vi "Load LVS.vi"(8 "error in (no error)":errorcluster, 10 "LVS Data (in)":T1={"Impulse Positions"=[], "No. Imp"=0, "Parameter Time Series"=[], "Parameter Impuls Series"=[], "Experiment Parameters"={"Freq"=0.0, "Vel"=0, "Acc"=0, "Stimulus"=""}, "Autosort File"=refnum, "Data File"={"Data Channels"=[], "Sample Rate"=0, "Channel List"=[]}, "Experiment data path"=path "/Macintosh HD/Users/patrick/Studium/Diploma Thesis/Data Analysis", "Image data path"=path "/Macintosh HD/Users/patrick/Studium/Diploma Thesis/Data Analysis", "LVS data path"=path "/Macintosh HD/Users/patrick/Studium/Diploma Thesis/Data Analysis", "Raw copy path"=path "/Macintosh HD/Users/patrick/Studium/Diploma Thesis/Data Analysis", "filename"="No file selected", "desaccading parameters"={"Tolerance"=0, "Acc Range"=0.0, "Sample Rate"=0, "Impulse Plane 2"=enum."Other", "Impulse dir"=FALSE}, "Experiment Parameters 2"={"Subject"="", "Strain"="", "Rotation plane"="", "Experimenter"="", "Trial"=0.0, "Time"=0.0}, "Excel"={"Excel._Application"=refnum, "Use Excel"=FALSE, "Worksheet SINE"=refnum, "Row SINE"=0, "Worksheet TRANS"=refnum, "Row TRANS"=0}, "Session Config File"=refnum, "Autosort Parameter Set"=1, "EMA Version"="", "desacc "={"Threshold 1 [Acc]"=7000.0, "Threshold 2 [% of TH1]"=60, "tolerance"=3, "Search WD "=0.1, " always use TH2"=FALSE, "Range"=2.0, "Max time"=120.0, "Min time"=20.0, "Velocity Threshold"=150}, "Cycle Nr for Saccades"={"POS"=0, "NEG"=0}, "calibration name"="No file selected"} {"Parameter Time Series"."time offset" format="%.3f"; "Parameter Time Series"."Gain" format="%.1f"; "Parameter Time Series"."Offset" format="%.1f"; "Parameter Time Series"."List 1" items=["Motor-Pos", "Motor-Vel", "Lx Position-in-Head", "Ly Position-in-Head", "Lz Position-in-Head", "Lx Velocity-in-Head", "Ly Velocity-in-Head", "Lz Velocity-in-Head", "Ll Velocity-in-Head", "Lr Velocity-in-Head", "Lx Accel-in-Head", "Ly Accel-in-Head", "Lz Accel-in-Head", "Rx Position-in-Head", "Ry Position-in-Head", "Rz Position-in-Head", "Rx Velocity-in-Head", "Ry Velocity-in-Head", "Rz Velocity-in-Head", "Rl Velocity-in-Head", "Rr Velocity-in-Head", "Rx Accel-in-Head", "Ry Accel-in-Head", "Rz Accel-in-Head", "Global Trigger", "", "", ""]; "Parameter Impuls Series"."Gain" format="%.1f"; "Parameter Impuls Series"."Offset" format="%.1f"}, 11 "Path (in)":path) -> (0 "error out":errorcluster, 2 "LVS Data (out)":T1={"Impulse Positions"=[], "No. Imp"=0, "Parameter Time Series"=[], "Parameter Impuls Series"=[], "Experiment Parameters"={"Freq"=0.0, "Vel"=0, "Acc"=0, "Stimulus"=""}, "Autosort File"=refnum, "Data File"={"Data Channels"=[], "Sample Rate"=0, "Channel List"=[]}, "Experiment data path"=path "/Macintosh HD/Users/patrick/Studium/Diploma Thesis/Data Analysis", "Image data path"=path "/Macintosh HD/Users/patrick/Studium/Diploma Thesis/Data Analysis", "LVS data path"=path "/Macintosh HD/Users/patrick/Studium/Diploma Thesis/Data Analysis", "Raw copy path"=path "/Macintosh HD/Users/patrick/Studium/Diploma Thesis/Data Analysis", "filename"="No file selected", "desaccading parameters"={"Tolerance"=0, "Acc Range"=0.0, "Sample Rate"=0, "Impulse Plane 2"=enum."Other", "Impulse dir"=FALSE}, "Experiment Parameters 2"={"Subject"="", "Strain"="", "Rotation plane"="", "Experimenter"="", "Trial"=0.0, "Time"=0.0}, "Excel"={"Excel._Application"=refnum, "Use Excel"=FALSE, "Worksheet SINE"=refnum, "Row SINE"=0, "Worksheet TRANS"=refnum, "Row TRANS"=0}, "Session Config File"=refnum, "Autosort Parameter Set"=1, "EMA Version"="", "desacc "={"Threshold 1 [Acc]"=7000.0, "Threshold 2 [% of TH1]"=60, "tolerance"=3, "Search WD "=0.1, " always use TH2"=FALSE, "Range"=2.0, "Max time"=120.0, "Min time"=20.0, "Velocity Threshold"=150}, "Cycle Nr for Saccades"={"POS"=0, "NEG"=0}, "calibration name"="No file selected"} {"Parameter Time Series"."time offset" format="%.3f"; "Parameter Time Series"."Gain" format="%.1f"; "Parameter Time Series"."Offset" format="%.1f"; "Parameter Time Series"."List 1" items=["Motor-Pos", "Motor-Vel", "Lx Position-in-Head", "Ly Position-in-Head", "Lz Position-in-Head", "Lx Velocity-in-Head", "Ly Velocity-in-Head", "Lz Velocity-in-Head", "Ll Velocity-in-Head", "Lr Velocity-in-Head", "Lx Accel-in-Head", "Ly Accel-in-Head", "Lz Accel-in-Head", "Rx Position-in-Head", "Ry Position-in-Head", "Rz Position-in-Head", "Rx Velocity-in-Head", "Ry Velocity-in-Head", "Rz Velocity-in-Head", "Rl Velocity-in-Head", "Rr Velocity-in-Head", "Rx Accel-in-Head", "Ry Accel-in-Head", "Rz Accel-in-Head", "Global Trigger", "", "", ""]; "Parameter Impuls Series"."Gain" format="%.1f"; "Parameter Impuls Series"."Offset" format="%.1f"}, 3 "Path (out)":path)   [LabVIEW 2016]
uses:
  type-defs/TD_Statemachine-Data.ctl
  type-defs/TD_Time Series.ctl
  type-defs/TD_Impulse Parameter.ctl
  core.lvlib
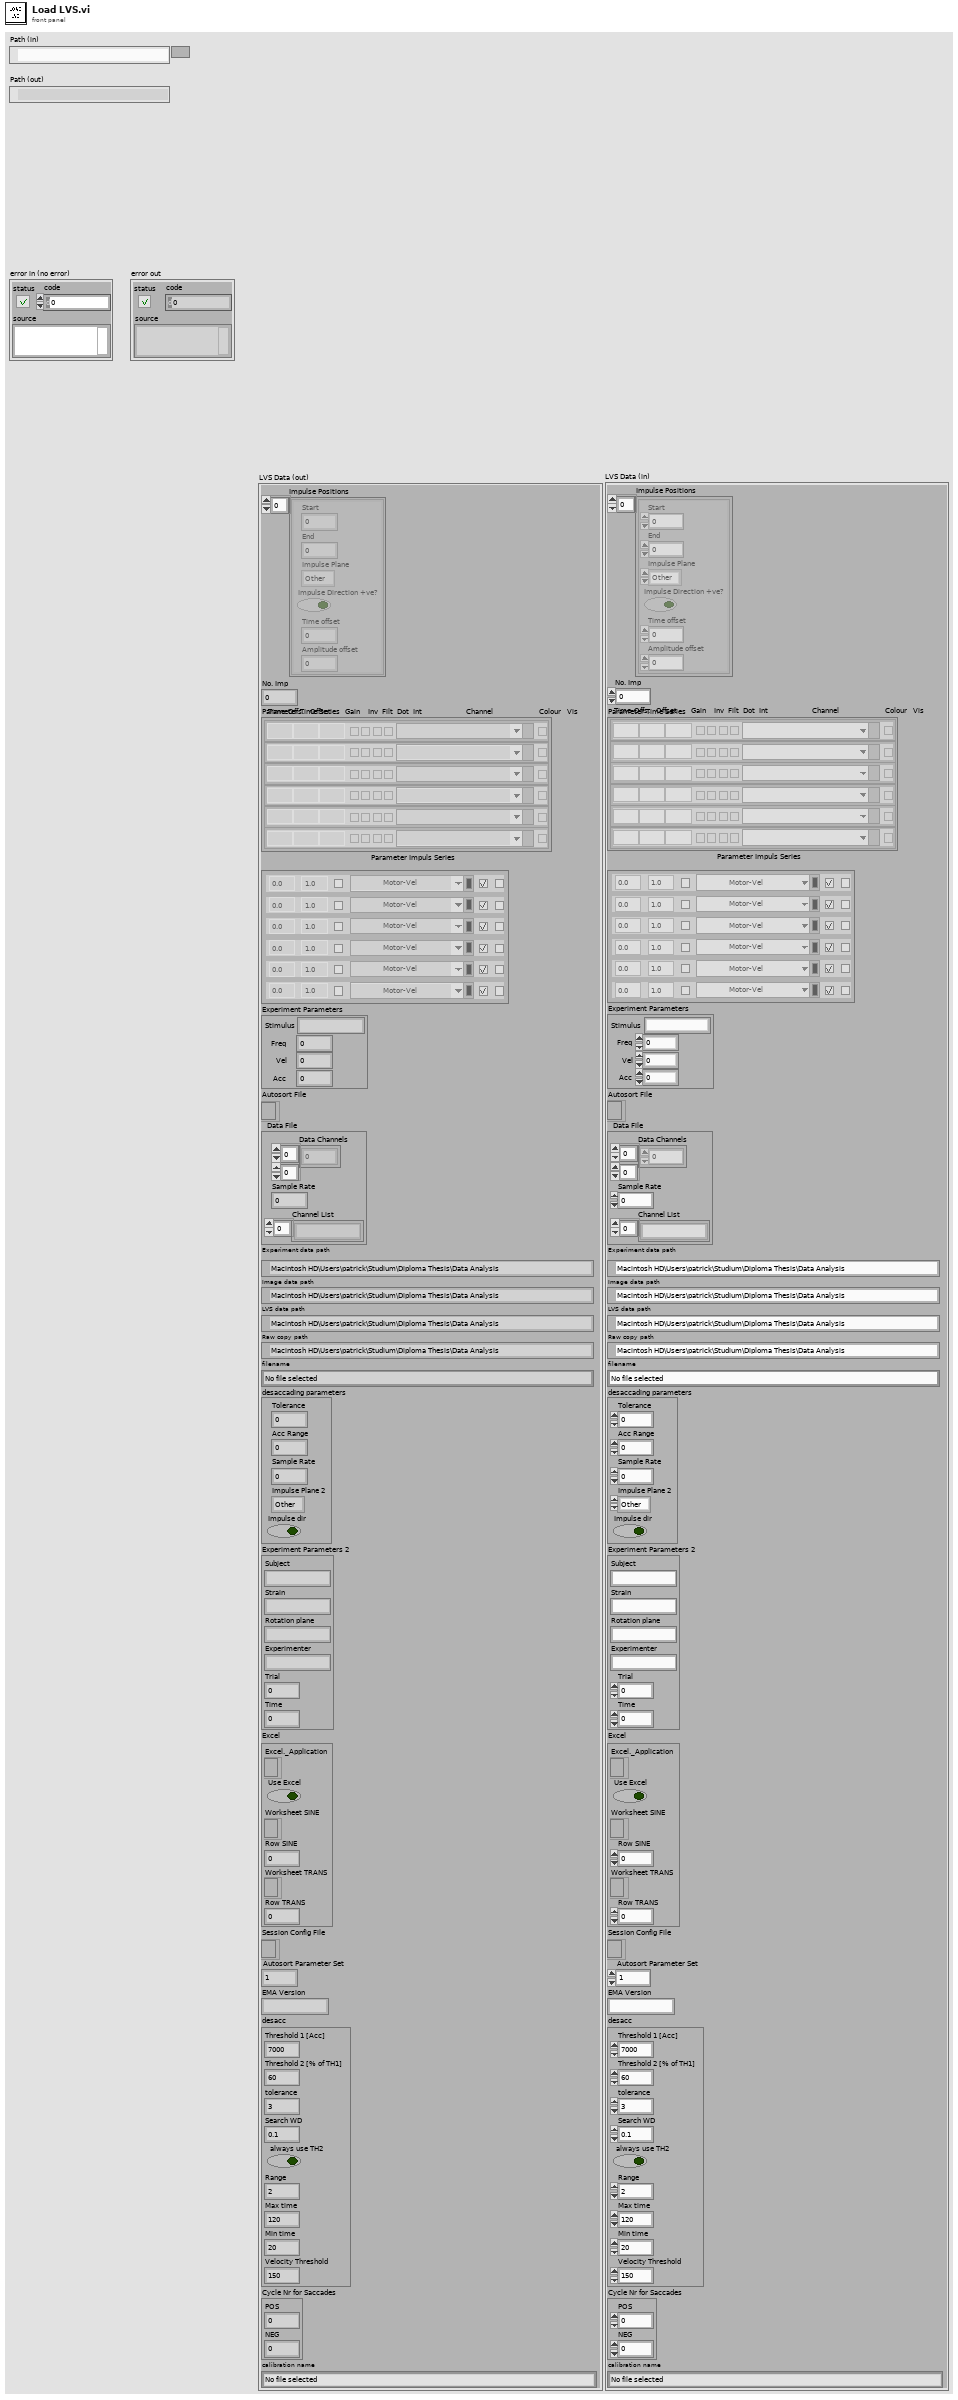
[diagram p1: front panel]
types:
  T1 = typedef "core.lvlib/TD_Statemachine-Data.ctl" = cluster{"Impulse Positions":cluster{"Start":i32, "End":i32, "Impulse Plane":enum16{"Other", "Yaw", "Pitch", "Roll", "LARP", "RALP"}, "Impulse Direction +ve?":bool, "Time offset":i32, "Amplitude offset":dbl}[], "No. Imp":i32, "Parameter Time Series":T2, "Parameter Impuls Series":T3, "Experiment Parameters":cluster{"Freq":dbl, "Vel":i32, "Acc":i32, "Stimulus":string}, "Autosort File":refnum<file>, "Data File":cluster{"Data Channels":dbl[][], "Sample Rate":i32, "Channel List":string[]}, "Experiment data path":path, "Image data path":path, "LVS data path":path, "Raw copy path":path, "filename":string, "desaccading parameters":cluster{"Tolerance":i32, "Acc Range":dbl, "Sample Rate":i32, "Impulse Plane 2":enum16{"Other", "Yaw", "Pitch", "Roll", "LARP", "RALP"}, "Impulse dir":bool}, "Experiment Parameters 2":cluster{"Subject":string, "Strain":string, "Rotation plane":string, "Experimenter":string, "Trial":dbl, "Time":dbl}, "Excel":cluster{"Excel._Application":refnum<k7>, "Use Excel":bool, "Worksheet SINE":refnum<k7>, "Row SINE":i32, "Worksheet TRANS":refnum<k7>, "Row TRANS":i32}, "Session Config File":refnum<file>, "Autosort Parameter Set":i32, "EMA Version":string, "desacc ":cluster{"Threshold 1 [Acc]":dbl, "Threshold 2 [% of TH1]":i32, "tolerance":i32, "Search WD ":dbl, " always use TH2":bool, "Range":dbl, "Max time":dbl, "Min time":dbl, "Velocity Threshold":i32}, "Cycle Nr for Saccades":cluster{"POS":i32, "NEG":i32}, "calibration name":string}
  T2 = typedef "core.lvlib/TD_Time Series.ctl" = cluster{"time offset":dbl, "Offset":dbl, "Gain":dbl, "inverse":bool, "filter data":bool, "dots":bool, "interpolate":bool, "List 1":u16, "Color Box":u32, "Boolean":bool}[]
  T3 = typedef "core.lvlib/TD_Impulse Parameter.ctl" = cluster{"Color":u32, "Visible":bool, "Channel":u16, "Invert":bool, "Desaccade":bool, "Offset":dbl, "Gain":dbl}[]
  T4 = cluster{"Data Channels":dbl[][], "Sample Rate":i32, "Channel List":string[]}
  T5 = cluster{"Freq":dbl, "Vel":i32, "Acc":i32, "Stimulus":string}
  T6 = cluster{"Subject":string, "Strain":string, "Rotation plane":string, "Experimenter":string, "Trial":dbl, "Time":dbl}
  T7 = cluster{"Impulse Positions":cluster{"Start":i32, "End":i32, "Impulse Plane":enum16{"Other", "Yaw", "Pitch", "Roll", "LARP", "RALP"}, "Impulse Direction +ve?":bool, "Time offset":i32, "Amplitude offset":dbl}[], "Old Impulse positions for Undo":cluster{"Start":i32, "End":i32, "Impulse Plane":enum16{"Other", "Yaw", "Pitch", "Roll", "LARP", "RALP"}, "Impulse Direction +ve?":bool, "Time offset":i32, "Amplitude offset":dbl}[], "No. Imp":i32}
  T8 = cluster{"\"Data File\" Cluster":cluster{"Data Channels":dbl[][], "Sample Rate":i32, "Channel List":string[]}, "OLD LVS Data Cluster":cluster{"Impulse Positions":cluster{"Start":i32, "End":i32, "Impulse Plane":enum16{"Other", "Yaw", "Pitch", "Roll", "LARP", "RALP"}, "Impulse Direction +ve?":bool, "Time offset":i32, "Amplitude offset":dbl}[], "Old Impulse positions for Undo":cluster{"Start":i32, "End":i32, "Impulse Plane":enum16{"Other", "Yaw", "Pitch", "Roll", "LARP", "RALP"}, "Impulse Direction +ve?":bool, "Time offset":i32, "Amplitude offset":dbl}[], "No. Imp":i32}}
  T9 = cluster{"Start":i32, "End":i32, "Impulse Plane":enum16{"Other", "Yaw", "Pitch", "Roll", "LARP", "RALP"}, "Impulse Direction +ve?":bool, "Time offset":i32, "Amplitude offset":dbl}[]
  T10 = cluster{"Impulse Positions":cluster{"Start":i32, "End":i32, "Impulse Plane":enum16{"Other", "Yaw", "Pitch", "Roll", "LARP", "RALP"}, "Impulse Direction +ve?":bool, "Time offset":i32, "Amplitude offset":dbl}[], "Old Impulse positions for Undo":cluster{"Start":i32, "End":i32, "Impulse Plane":enum16{"Other", "Yaw", "Pitch", "Roll", "LARP", "RALP"}, "Impulse Direction +ve?":bool, "Time offset":i32, "Amplitude offset":dbl}[], "No. Imp":i32, "Parameter Time Series":T2, "Parameter Impuls Series":T3, "Experiment Parameters":cluster{"Freq":dbl, "Vel":i32, "Acc":i32, "Stimulus":string}, "Autosort File":refnum<file>, "Data File":cluster{"Data Channels":dbl[][], "Sample Rate":i32, "Channel List":string[]}, "Experiment data path":path, "Image data path":path, "LVS data path":path, "Raw copy path":path, "filename":string, "desaccading parameters":cluster{"Tolerance":i32, "Acc Range":dbl, "Sample Rate":i32, "Impulse Plane 2":enum16{"Other", "Yaw", "Pitch", "Roll", "LARP", "RALP"}, "Impulse dir":bool}, "Experiment Parameters 2":cluster{"Subject":string, "Strain":string, "Rotation plane":string, "Experimenter":string, "Trial":dbl, "Time":dbl}, "Excel":cluster{"Excel._Application":refnum<k7>, "Use Excel":bool, "Worksheet SINE":refnum<k7>, "Row SINE":i32, "Worksheet TRANS":refnum<k7>, "Row TRANS":i32}, "Session Config File":refnum<file>, "Autosort Parameter Set":i32, "EMA Version":string, "desacc ":cluster{"Threshold 1 [Acc]":dbl, "Threshold 2 [% of TH1]":i32, "tolerance":i32, "Search WD ":dbl, " always use TH2":bool, "Range":dbl, "Max time":dbl, "Min time":dbl}}
  T11 = cluster{"\"Data File\" Cluster":cluster{"Data Channels":dbl[][], "Sample Rate":i32, "Channel List":string[]}, "EMA 2011a Data Cluster":cluster{"Impulse Positions":cluster{"Start":i32, "End":i32, "Impulse Plane":enum16{"Other", "Yaw", "Pitch", "Roll", "LARP", "RALP"}, "Impulse Direction +ve?":bool, "Time offset":i32, "Amplitude offset":dbl}[], "Old Impulse positions for Undo":cluster{"Start":i32, "End":i32, "Impulse Plane":enum16{"Other", "Yaw", "Pitch", "Roll", "LARP", "RALP"}, "Impulse Direction +ve?":bool, "Time offset":i32, "Amplitude offset":dbl}[], "No. Imp":i32, "Parameter Time Series":T2, "Parameter Impuls Series":T3, "Experiment Parameters":cluster{"Freq":dbl, "Vel":i32, "Acc":i32, "Stimulus":string}, "Autosort File":refnum<file>, "Data File":cluster{"Data Channels":dbl[][], "Sample Rate":i32, "Channel List":string[]}, "Experiment data path":path, "Image data path":path, "LVS data path":path, "Raw copy path":path, "filename":string, "desaccading parameters":cluster{"Tolerance":i32, "Acc Range":dbl, "Sample Rate":i32, "Impulse Plane 2":enum16{"Other", "Yaw", "Pitch", "Roll", "LARP", "RALP"}, "Impulse dir":bool}, "Experiment Parameters 2":cluster{"Subject":string, "Strain":string, "Rotation plane":string, "Experimenter":string, "Trial":dbl, "Time":dbl}, "Excel":cluster{"Excel._Application":refnum<k7>, "Use Excel":bool, "Worksheet SINE":refnum<k7>, "Row SINE":i32, "Worksheet TRANS":refnum<k7>, "Row TRANS":i32}, "Session Config File":refnum<file>, "Autosort Parameter Set":i32, "EMA Version":string, "desacc ":cluster{"Threshold 1 [Acc]":dbl, "Threshold 2 [% of TH1]":i32, "tolerance":i32, "Search WD ":dbl, " always use TH2":bool, "Range":dbl, "Max time":dbl, "Min time":dbl}}}
  T12 = cluster{"Tolerance":i32, "Acc Range":dbl, "Sample Rate":i32, "Impulse Plane 2":enum16{"Other", "Yaw", "Pitch", "Roll", "LARP", "RALP"}, "Impulse dir":bool}
  T13 = cluster{"Impulse Positions":cluster{"Start":i32, "End":i32, "Impulse Plane":enum16{"Other", "Yaw", "Pitch", "Roll", "LARP", "RALP"}, "Impulse Direction +ve?":bool, "Time offset":i32, "Amplitude offset":dbl}[], "Old Impulse positions for Undo":cluster{"Start":i32, "End":i32, "Impulse Plane":enum16{"Other", "Yaw", "Pitch", "Roll", "LARP", "RALP"}, "Impulse Direction +ve?":bool, "Time offset":i32, "Amplitude offset":dbl}[][], "No. Imp":i32, "Parameter Time Series":T2, "Parameter Impuls Series":T3, "Experiment Parameters":cluster{"Freq":dbl, "Vel":i32, "Acc":i32, "Stimulus":string}, "Autosort File":refnum<file>, "Data File":cluster{"Data Channels":dbl[][], "Sample Rate":i32, "Channel List":string[]}, "Experiment data path":path, "Image data path":path, "LVS data path":path, "Raw copy path":path, "filename":string, "desaccading parameters":cluster{"Tolerance":i32, "Acc Range":dbl, "Sample Rate":i32, "Impulse Plane 2":enum16{"Other", "Yaw", "Pitch", "Roll", "LARP", "RALP"}, "Impulse dir":bool}, "Experiment Parameters 2":cluster{"Subject":string, "Strain":string, "Rotation plane":string, "Experimenter":string, "Trial":dbl, "Time":dbl}, "Excel":cluster{"Excel._Application":refnum<k7>, "Use Excel":bool, "Worksheet SINE":refnum<k7>, "Row SINE":i32, "Worksheet TRANS":refnum<k7>, "Row TRANS":i32}, "Session Config File":refnum<file>, "Autosort Parameter Set":i32, "EMA Version":string, "desacc ":cluster{"Threshold 1 [Acc]":dbl, "Threshold 2 [% of TH1]":i32, "tolerance":i32, "Search WD ":dbl, " always use TH2":bool, "Range":dbl, "Max time":dbl, "Min time":dbl, "Velocity Threshold":i32}, "Cycle Nr for Saccades":cluster{"POS":i32, "NEG":i32}, "Undo Counter":i32, "History Length":i32, "Redo Counter":i32, "Histpry Position":i32, "Raw Data File":cluster{"Data Channels":dbl[][], "Sample Rate":i32, "Channel List":string[]}}
  T14 = cluster{"\"Data File\" Cluster":cluster{"Data Channels":dbl[][], "Sample Rate":i32, "Channel List":string[]}, "EMA 2011b Data Cluster":cluster{"Impulse Positions":cluster{"Start":i32, "End":i32, "Impulse Plane":enum16{"Other", "Yaw", "Pitch", "Roll", "LARP", "RALP"}, "Impulse Direction +ve?":bool, "Time offset":i32, "Amplitude offset":dbl}[], "Old Impulse positions for Undo":cluster{"Start":i32, "End":i32, "Impulse Plane":enum16{"Other", "Yaw", "Pitch", "Roll", "LARP", "RALP"}, "Impulse Direction +ve?":bool, "Time offset":i32, "Amplitude offset":dbl}[][], "No. Imp":i32, "Parameter Time Series":T2, "Parameter Impuls Series":T3, "Experiment Parameters":cluster{"Freq":dbl, "Vel":i32, "Acc":i32, "Stimulus":string}, "Autosort File":refnum<file>, "Data File":cluster{"Data Channels":dbl[][], "Sample Rate":i32, "Channel List":string[]}, "Experiment data path":path, "Image data path":path, "LVS data path":path, "Raw copy path":path, "filename":string, "desaccading parameters":cluster{"Tolerance":i32, "Acc Range":dbl, "Sample Rate":i32, "Impulse Plane 2":enum16{"Other", "Yaw", "Pitch", "Roll", "LARP", "RALP"}, "Impulse dir":bool}, "Experiment Parameters 2":cluster{"Subject":string, "Strain":string, "Rotation plane":string, "Experimenter":string, "Trial":dbl, "Time":dbl}, "Excel":cluster{"Excel._Application":refnum<k7>, "Use Excel":bool, "Worksheet SINE":refnum<k7>, "Row SINE":i32, "Worksheet TRANS":refnum<k7>, "Row TRANS":i32}, "Session Config File":refnum<file>, "Autosort Parameter Set":i32, "EMA Version":string, "desacc ":cluster{"Threshold 1 [Acc]":dbl, "Threshold 2 [% of TH1]":i32, "tolerance":i32, "Search WD ":dbl, " always use TH2":bool, "Range":dbl, "Max time":dbl, "Min time":dbl, "Velocity Threshold":i32}, "Cycle Nr for Saccades":cluster{"POS":i32, "NEG":i32}, "Undo Counter":i32, "History Length":i32, "Redo Counter":i32, "Histpry Position":i32, "Raw Data File":cluster{"Data Channels":dbl[][], "Sample Rate":i32, "Channel List":string[]}}}
  T15 = cluster{"Threshold 1 [Acc]":dbl, "Threshold 2 [% of TH1]":i32, "tolerance":i32, "Search WD ":dbl, " always use TH2":bool, "Range":dbl, "Max time":dbl, "Min time":dbl, "Velocity Threshold":i32}
  T16 = cluster{"Impulse Positions":cluster{"Start":i32, "End":i32, "Impulse Plane":enum16{"Other", "Yaw", "Pitch", "Roll", "LARP", "RALP"}, "Impulse Direction +ve?":bool, "Time offset":i32, "Amplitude offset":dbl}[], "Old Impulse positions for Undo":cluster{"Start":i32, "End":i32, "Impulse Plane":enum16{"Other", "Yaw", "Pitch", "Roll", "LARP", "RALP"}, "Impulse Direction +ve?":bool, "Time offset":i32, "Amplitude offset":dbl}[][], "No. Imp":i32, "Parameter Time Series":T2, "Parameter Impuls Series":T3, "Experiment Parameters":cluster{"Freq":dbl, "Vel":i32, "Acc":i32, "Stimulus":string}, "Autosort File":refnum<file>, "Data File":cluster{"Data Channels":dbl[][], "Sample Rate":i32, "Channel List":string[]}, "Experiment data path":path, "Image data path":path, "LVS data path":path, "Raw copy path":path, "filename":string, "desaccading parameters":cluster{"Tolerance":i32, "Acc Range":dbl, "Sample Rate":i32, "Impulse Plane 2":enum16{"Other", "Yaw", "Pitch", "Roll", "LARP", "RALP"}, "Impulse dir":bool}, "Experiment Parameters 2":cluster{"Subject":string, "Strain":string, "Rotation plane":string, "Experimenter":string, "Trial":dbl, "Time":dbl}, "Excel":cluster{"Excel._Application":refnum<k7>, "Use Excel":bool, "Worksheet SINE":refnum<k7>, "Row SINE":i32, "Worksheet TRANS":refnum<k7>, "Row TRANS":i32}, "Session Config File":refnum<file>, "Autosort Parameter Set":i32, "EMA Version":string, "desacc ":cluster{"Threshold 1 [Acc]":dbl, "Threshold 2 [% of TH1]":i32, "tolerance":i32, "Search WD ":dbl, " always use TH2":bool, "Range":dbl, "Max time":dbl, "Min time":dbl, "Velocity Threshold":i32}, "Cycle Nr for Saccades":cluster{"POS":i32, "NEG":i32}, "Undo Counter":i32, "History Length":i32, "Redo Counter":i32, "Histpry Position":i32, "Raw Data File":cluster{"Data Channels":dbl[][], "Sample Rate":i32, "Channel List":string[]}, "calibration name":string}
  T17 = cluster{"\"Data File\" Cluster":cluster{"Data Channels":dbl[][], "Sample Rate":i32, "Channel List":string[]}, "EMA 2016a Data Cluster":cluster{"Impulse Positions":cluster{"Start":i32, "End":i32, "Impulse Plane":enum16{"Other", "Yaw", "Pitch", "Roll", "LARP", "RALP"}, "Impulse Direction +ve?":bool, "Time offset":i32, "Amplitude offset":dbl}[], "Old Impulse positions for Undo":cluster{"Start":i32, "End":i32, "Impulse Plane":enum16{"Other", "Yaw", "Pitch", "Roll", "LARP", "RALP"}, "Impulse Direction +ve?":bool, "Time offset":i32, "Amplitude offset":dbl}[][], "No. Imp":i32, "Parameter Time Series":T2, "Parameter Impuls Series":T3, "Experiment Parameters":cluster{"Freq":dbl, "Vel":i32, "Acc":i32, "Stimulus":string}, "Autosort File":refnum<file>, "Data File":cluster{"Data Channels":dbl[][], "Sample Rate":i32, "Channel List":string[]}, "Experiment data path":path, "Image data path":path, "LVS data path":path, "Raw copy path":path, "filename":string, "desaccading parameters":cluster{"Tolerance":i32, "Acc Range":dbl, "Sample Rate":i32, "Impulse Plane 2":enum16{"Other", "Yaw", "Pitch", "Roll", "LARP", "RALP"}, "Impulse dir":bool}, "Experiment Parameters 2":cluster{"Subject":string, "Strain":string, "Rotation plane":string, "Experimenter":string, "Trial":dbl, "Time":dbl}, "Excel":cluster{"Excel._Application":refnum<k7>, "Use Excel":bool, "Worksheet SINE":refnum<k7>, "Row SINE":i32, "Worksheet TRANS":refnum<k7>, "Row TRANS":i32}, "Session Config File":refnum<file>, "Autosort Parameter Set":i32, "EMA Version":string, "desacc ":cluster{"Threshold 1 [Acc]":dbl, "Threshold 2 [% of TH1]":i32, "tolerance":i32, "Search WD ":dbl, " always use TH2":bool, "Range":dbl, "Max time":dbl, "Min time":dbl, "Velocity Threshold":i32}, "Cycle Nr for Saccades":cluster{"POS":i32, "NEG":i32}, "Undo Counter":i32, "History Length":i32, "Redo Counter":i32, "Histpry Position":i32, "Raw Data File":cluster{"Data Channels":dbl[][], "Sample Rate":i32, "Channel List":string[]}, "calibration name":string}}
  T18 = cluster{"Impulse Positions":cluster{"Start":i32, "End":i32, "Impulse Plane":enum16{"Other", "Yaw", "Pitch", "Roll", "LARP", "RALP"}, "Impulse Direction +ve?":bool, "Time offset":i32, "Amplitude offset":dbl}[], "No. Imp":i32, "Parameter Time Series":T2, "Parameter Impuls Series":T3, "Experiment Parameters":cluster{"Freq":dbl, "Vel":i32, "Acc":i32, "Stimulus":string}, "Autosort File":refnum<file>, "Data File":cluster{"Data Channels":dbl[][], "Sample Rate":i32, "Channel List":string[]}, "Experiment data path":path, "Image data path":path, "LVS data path":path, "Raw copy path":path, "filename":string, "desaccading parameters":cluster{"Tolerance":i32, "Acc Range":dbl, "Sample Rate":i32, "Impulse Plane 2":enum16{"Other", "Yaw", "Pitch", "Roll", "LARP", "RALP"}, "Impulse dir":bool}, "Experiment Parameters 2":cluster{"Subject":string, "Strain":string, "Rotation plane":string, "Experimenter":string, "Trial":dbl, "Time":dbl}, "Excel":cluster{"Excel._Application":refnum<k7>, "Use Excel":bool, "Worksheet SINE":refnum<k7>, "Row SINE":i32, "Worksheet TRANS":refnum<k7>, "Row TRANS":i32}, "Session Config File":refnum<file>, "Autosort Parameter Set":i32, "EMA Version":string, "desacc ":cluster{"Threshold 1 [Acc]":dbl, "Threshold 2 [% of TH1]":i32, "tolerance":i32, "Search WD ":dbl, " always use TH2":bool, "Range":dbl, "Max time":dbl, "Min time":dbl, "Velocity Threshold":i32}, "Cycle Nr for Saccades":cluster{"POS":i32, "NEG":i32}, "calibration name":string}
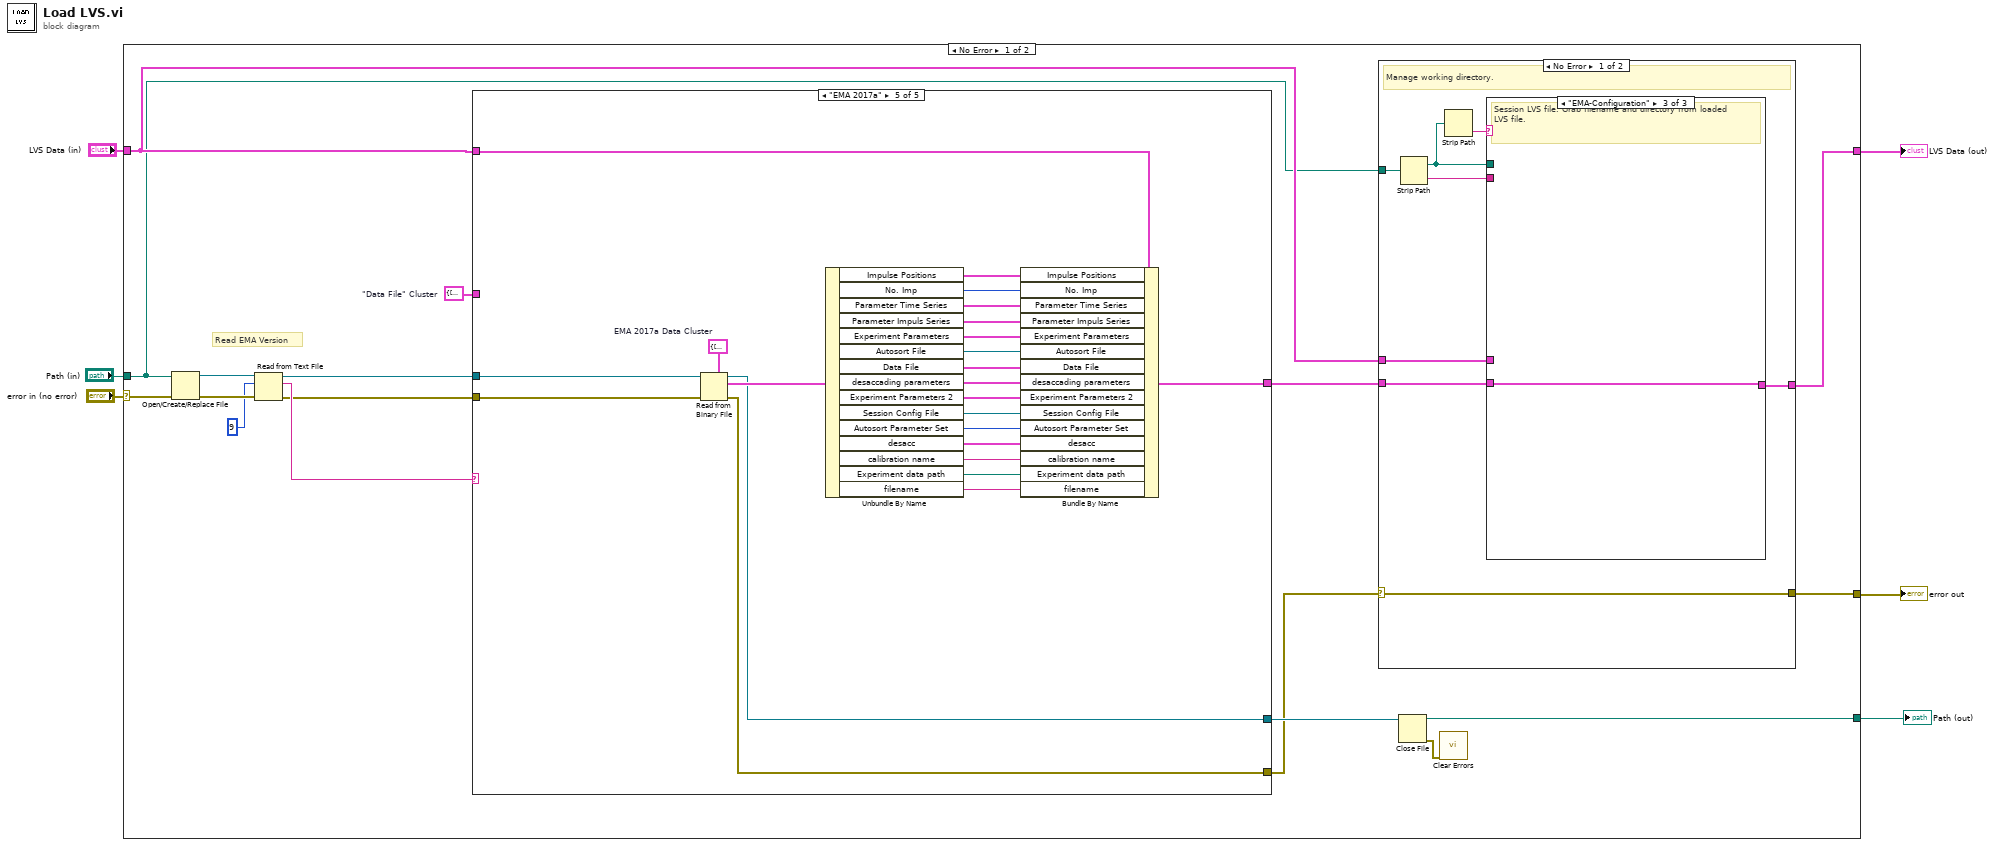
[diagram p0: block diagram]
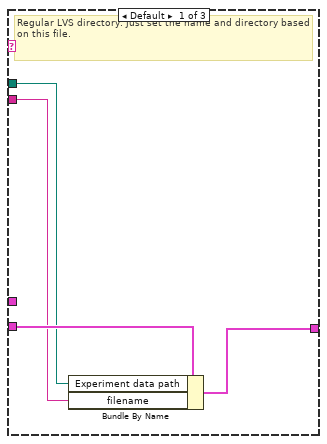
[diagram p2: hidden frame]
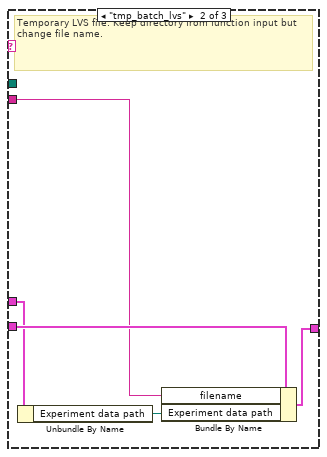
[diagram p3: hidden frame]
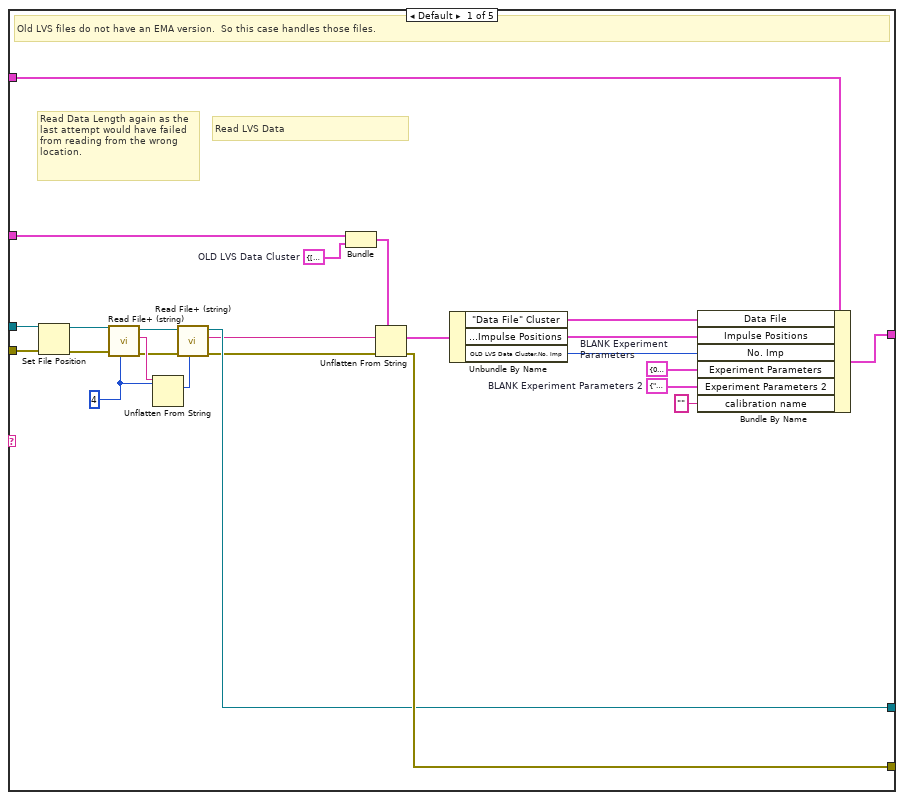
[diagram p5: hidden frame]
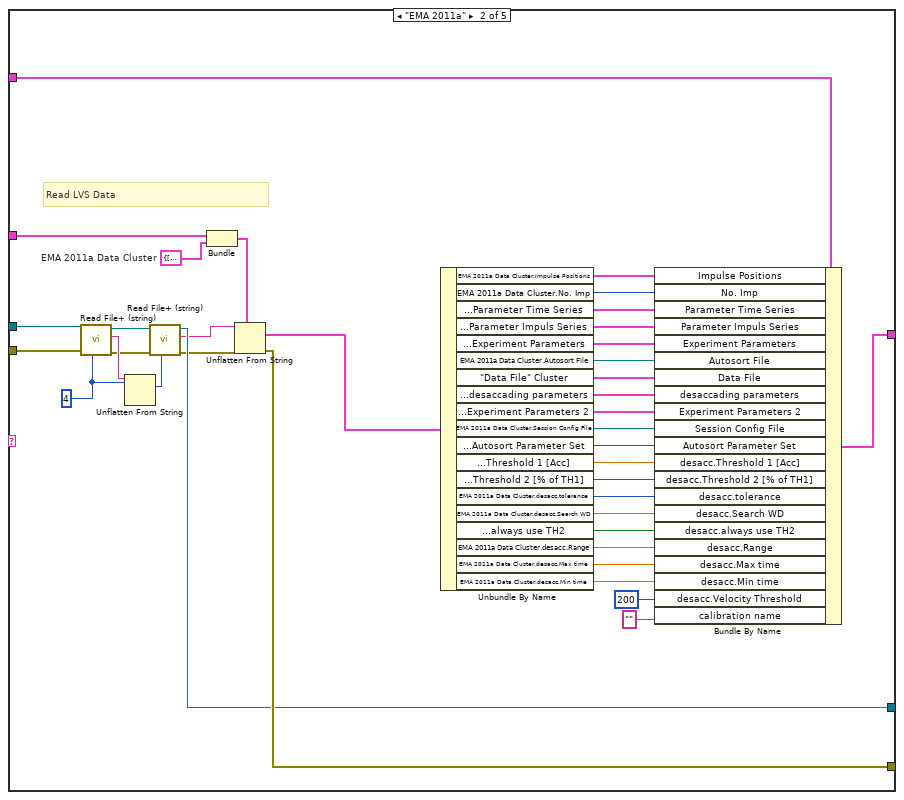
[diagram p6: hidden frame]
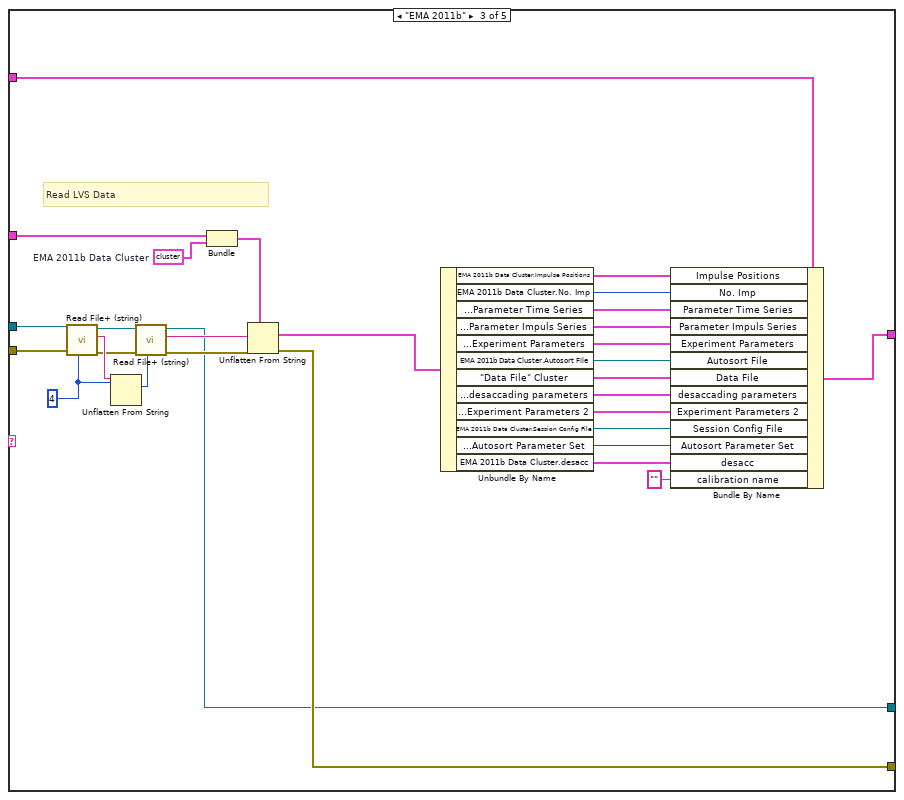
[diagram p7: hidden frame]
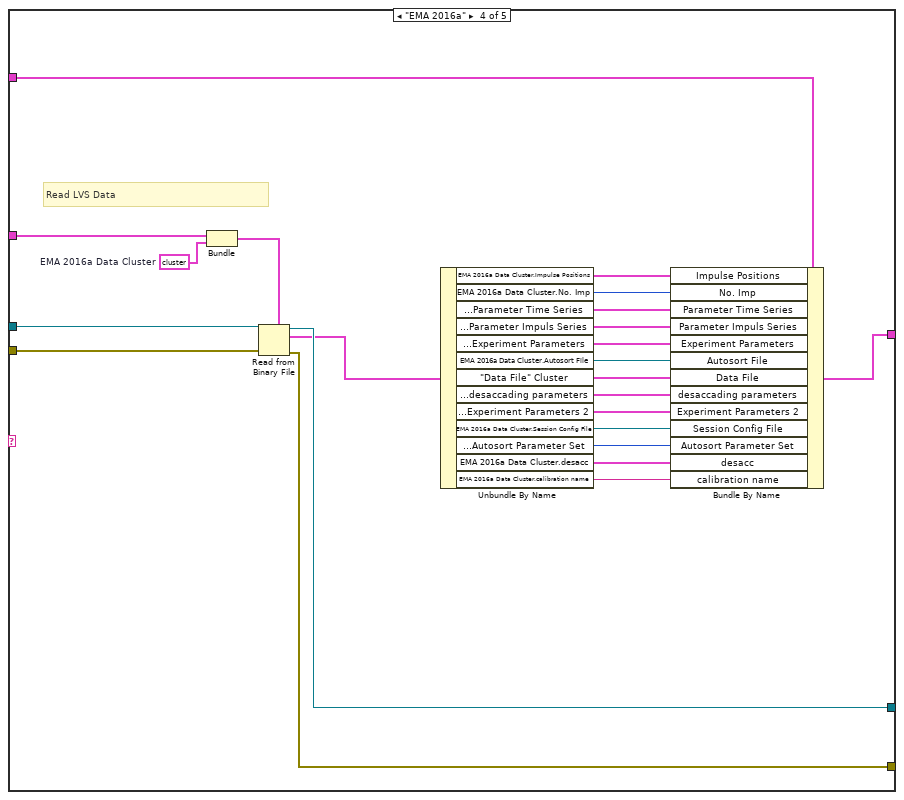
[diagram p8: hidden frame]
diagram:
  n1 = case shown="No Error" "error in (no error)" {
    selector: "error in (no error)" -> [w23 w184]
    tunnel: "Path (in)" -> [w9 w185]
    tunnel: [w15 w185] -> w4
    tunnel: [w7 w184] -> w3
    tunnel: [w8 w183] -> w2
    tunnel: "LVS Data (in)" -> [w10 w183]
    frame No Error {
      w18 = T4 {"Data Channels"=[], "Sample Rate"=0, "Channel List"=[]}  # "Data File" Cluster
      # "Read EMA Version"
      n2 = Open/Create/Replace File(file path (use dialog)=w9, error in=w23) -> (refnum out=w22:refnum<file>, error out=w21:errorcluster)  [unwired: 4 in, 1 out]
      n3 = Read from Text File(file (use dialog)=w22, count=9, error in=w21) -> (refnum out=w13:refnum<file>, text=w19:string, error out=w14:errorcluster)  [unwired: 1 in, 1 out]
      n4 = case shown="\"EMA 2017a\"" w19 {
        tunnel: w13 -> [w67 w73 w117 w142 w182]
        tunnel: w14 -> [w68 w72 w116 w141 w181]
        tunnel: w10 -> [w64 w102 w135 w158 w179]
        tunnel: [w57 w101 w134 w157 w178] -> w11
        tunnel: [w56 w103 w109 w139 w163] -> w12
        tunnel: [w46 w71 w108 w140 w164] -> w17
        tunnel: w18 -> [w55 w106 w136 w159 _]
        frame Default {
          w52 = 4 ("count")
          w59 = T5 {"Freq"=0.0, "Vel"=0, "Acc"=0, "Stimulus"=""}  # BLANK Experiment Parameters
          w58 = T6 {"Subject"="", "Strain"="", "Rotation plane"="", "Experimenter"="", "Trial"=0.0, "Time"=0.0}  # BLANK Experiment Parameters 2
          w66 = T7 {"Impulse Positions"=[], "Old Impulse positions for Undo"=[], "No. Imp"=0}  # OLD LVS Data Cluster
          # "Read LVS Data"
          # "Read Data Length again as the last attempt would have failed from reading from the wrong location."
          # "Old LVS files do not have an EMA version.  So this case handles those files."
          n5 = Set File Position(refnum=w67, error in=w68) -> (refnum out=w48:refnum<file>, error out=w47:errorcluster)  [unwired: 2 in]
          n6 = call <vilib>:"Read File+ (string).vi"("count"=w52, "error in (no error)"=w47, "refnum"=w48) -> ("error out"=w49:errorcluster, "string"=w51:string, "dup refnum"=w50:refnum<file>)  [unwired: 4 in, 2 out]
          n7 = Unflatten From String(type=w52, binary string=w51) -> (value=w53:i32)  [unwired: 3 in, 2 out]
          n8 = call <vilib>:"Read File+ (string).vi"("count"=w53, "error in (no error)"=w49, "refnum"=w50) -> ("error out"=w45:errorcluster, "string"=w44:string, "dup refnum"=w46:refnum<file>)  [unwired: 4 in, 2 out]
          n9 = Bundle("\"Data File\" Cluster"=w55, "OLD LVS Data Cluster"=w66) -> (w65:T8)  [unwired: 1 in]
          n10 = Unflatten From String(type=w65, binary string=w44, error in (no error)=w45) -> (value=w63:T8, error out=w56:errorcluster)  [unwired: 2 in, 1 out]
          n11 = Unbundle By Name(w63) -> ("\"Data File\" Cluster"=w62:T4, "OLD LVS Data Cluster.Impulse Positions"=w61:T9, "OLD LVS Data Cluster.No. Imp"=w60:i32)
          n12 = Bundle By Name(cluster=w64, "Data File"=w62, "Impulse Positions"=w61, "No. Imp"=w60, "Experiment Parameters"=w59, "Experiment Parameters 2"=w58, "calibration name"="") -> (w57:T1)
        }
        frame "EMA 2011a" {
          w77 = 4 ("count")
          w105 = T10 {"Impulse Positions"=[], "Old Impulse positions for Undo"=[], "No. Imp"=0, "Parameter Time Series"=[], "Parameter Impuls Series"=[], "Experiment Parameters"={"Freq"=0.0, "Vel"=0, "Acc"=0, "Stimulus"=""}, "Autosort File"=refnum, "Data File"={"Data Channels"=[], "Sample Rate"=0, "Channel List"=[]}, "Experiment data path"=path "/Macintosh HD/Users/patrick/Studium/Diploma Thesis/Data Analysis", "Image data path"=path "/Macintosh HD/Users/patrick/Studium/Diploma Thesis/Data Analysis", "LVS data path"=path "/Macintosh HD/Users/patrick/Studium/Diploma Thesis/Data Analysis", "Raw copy path"=path "/Macintosh HD/Users/patrick/Studium/Diploma Thesis/Data Analysis", "filename"="No file selected", "desaccading parameters"={"Tolerance"=0, "Acc Range"=0.0, "Sample Rate"=0, "Impulse Plane 2"=enum."Other", "Impulse dir"=FALSE}, "Experiment Parameters 2"={"Subject"="", "Strain"="", "Rotation plane"="", "Experimenter"="", "Trial"=0.0, "Time"=0.0}, "Excel"={"Excel._Application"=refnum, "Use Excel"=FALSE, "Worksheet SINE"=refnum, "Row SINE"=0, "Worksheet TRANS"=refnum, "Row TRANS"=0}, "Session Config File"=refnum, "Autosort Parameter Set"=1, "EMA Version"="", "desacc "={"Threshold 1 [Acc]"=1617.080808080808, "Threshold 2 [% of TH1]"=67, "tolerance"=5, "Search WD "=0.19090909090909092, " always use TH2"=TRUE, "Range"=3.2323232323232323, "Max time"=200.0, "Min time"=20.0}}  # EMA 2011a Data Cluster
          # "Read LVS Data"
          n13 = call <vilib>:"Read File+ (string).vi"("count"=w77, "error in (no error)"=w72, "refnum"=w73) -> ("error out"=w74:errorcluster, "string"=w76:string, "dup refnum"=w75:refnum<file>)  [unwired: 4 in, 2 out]
          n14 = Unflatten From String(type=w77, binary string=w76) -> (value=w78:i32)  [unwired: 3 in, 2 out]
          n15 = call <vilib>:"Read File+ (string).vi"("count"=w78, "error in (no error)"=w74, "refnum"=w75) -> ("error out"=w70:errorcluster, "string"=w69:string, "dup refnum"=w71:refnum<file>)  [unwired: 4 in, 2 out]
          n16 = Bundle("\"Data File\" Cluster"=w106, "EMA 2011a Data Cluster"=w105) -> (w104:T11)  [unwired: 1 in]
          n17 = Unflatten From String(type=w104, binary string=w69, error in (no error)=w70) -> (value=w80:T11, error out=w103:errorcluster)  [unwired: 2 in, 1 out]
          n18 = Unbundle By Name(w80) -> ("EMA 2011a Data Cluster.Impulse Positions"=w99:T9, "EMA 2011a Data Cluster.No. Imp"=w98:i32, "EMA 2011a Data Cluster.Parameter Time Series"=w97:T2, "EMA 2011a Data Cluster.Parameter Impuls Series"=w96:T3, "EMA 2011a Data Cluster.Experiment Parameters"=w95:T5, "EMA 2011a Data Cluster.Autosort File"=w94:refnum<file>, "\"Data File\" Cluster"=w93:T4, "EMA 2011a Data Cluster.desaccading parameters"=w92:T12, "EMA 2011a Data Cluster.Experiment Parameters 2"=w91:T6, "EMA 2011a Data Cluster.Session Config File"=w90:refnum<file>, "EMA 2011a Data Cluster.Autosort Parameter Set"=w89:i32, "EMA 2011a Data Cluster.desacc.Threshold 1 [Acc]"=w88:dbl, "EMA 2011a Data Cluster.desacc.Threshold 2 [% of TH1]"=w87:i32, "EMA 2011a Data Cluster.desacc.tolerance"=w86:i32, "EMA 2011a Data Cluster.desacc.Search WD"=w85:dbl, "EMA 2011a Data Cluster.desacc.always use TH2"=w84:bool, "EMA 2011a Data Cluster.desacc.Range"=w83:dbl, "EMA 2011a Data Cluster.desacc.Max time"=w82:dbl, "EMA 2011a Data Cluster.desacc.Min time"=w81:dbl)
          n19 = Bundle By Name(cluster=w102, "Impulse Positions"=w99, "No. Imp"=w98, "Parameter Time Series"=w97, "Parameter Impuls Series"=w96, "Experiment Parameters"=w95, "Autosort File"=w94, "Data File"=w93, "desaccading parameters"=w92, "Experiment Parameters 2"=w91, "Session Config File"=w90, "Autosort Parameter Set"=w89, "desacc.Threshold 1 [Acc]"=w88, "desacc.Threshold 2 [% of TH1]"=w87, "desacc.tolerance"=w86, "desacc.Search WD"=w85, "desacc.always use TH2"=w84, "desacc.Range"=w83, "desacc.Max time"=w82, "desacc.Min time"=w81, "desacc.Velocity Threshold"=200 ("desacc .Velocity Threshold"), "calibration name"="") -> (w101:T1)
        }
        frame "EMA 2011b" {
          w119 = 4 ("count")
          w122 = T13 {"Impulse Positions"=[{"Start"=4942, "End"=5034, "Impulse Plane"=enum."Yaw", "Impulse Direction +ve?"=TRUE, "Time offset"=0, "Amplitude offset"=0.0}, {"Start"=5524, "End"=5615, "Impulse Plane"=enum."Yaw", "Impulse Direction +ve?"=FALSE, "Time offset"=0, "Amplitude offset"=0.0}, {"Start"=6320, "End"=6414, "Impulse Plane"=enum."Yaw", "Impulse Direction +ve?"=FALSE, "Time offset"=0, "Amplitude offset"=0.0}, {"Start"=6789, "End"=6880, "Impulse Plane"=enum."Yaw", "Impulse Direction +ve?"=TRUE, "Time offset"=0, "Amplitude offset"=0.0}, {"Start"=7275, "End"=7365, "Impulse Plane"=enum."Yaw", "Impulse Direction +ve?"=FALSE, "Time offset"=0, "Amplitude offset"=0.0}, {"Start"=7765, "End"=7854, "Impulse Plane"=enum."Yaw", "Impulse Direction +ve?"=FALSE, "Time offset"=0, "Amplitude offset"=0.0}, {"Start"=8262, "End"=8354, "Impulse Plane"=enum."Yaw", "Impulse Direction +ve?"=TRUE, "Time offset"=0, "Amplitude offset"=0.0}, {"Start"=9102, "End"=9192, "Impulse Plane"=enum."Yaw", "Impulse Direction +ve?"=TRUE, "Time offset"=0, "Amplitude offset"=0.0}, {"Start"=9641, "End"=9736, "Impulse Plane"=enum."Yaw", "Impulse Direction +ve?"=FALSE, "Time offset"=0, "Amplitude offset"=0.0}, {"Start"=10150, "End"=10242, "Impulse Plane"=enum."Yaw", "Impulse Direction +ve?"=FALSE, "Time offset"=0, "Amplitude offset"=0.0}, {"Start"=10613, "End"=10703, "Impulse Plane"=enum."Yaw", "Impulse Direction +ve?"=TRUE, "Time offset"=0, "Amplitude offset"=0.0}, {"Start"=11147, "End"=11237, "Impulse Plane"=enum."Yaw", "Impulse Direction +ve?"=TRUE, "Time offset"=0, "Amplitude offset"=0.0}, {"Start"=11689, "End"=11781, "Impulse Plane"=enum."Yaw", "Impulse Direction +ve?"=TRUE, "Time offset"=0, "Amplitude offset"=0.0}, {"Start"=12321, "End"=12416, "Impulse Plane"=enum."Yaw", "Impulse Direction +ve?"=FALSE, "Time offset"=0, "Amplitude offset"=0.0}, {"Start"=12810, "End"=12901, "Impulse Plane"=enum."Yaw", "Impulse Direction +ve?"=FALSE, "Time offset"=0, "Amplitude offset"=0.0}, {"Start"=13306, "End"=13397, "Impulse Plane"=enum."Yaw", "Impulse Direction +ve?"=FALSE, "Time offset"=0, "Amplitude offset"=0.0}, {"Start"=13888, "End"=13980, "Impulse Plane"=enum."Yaw", "Impulse Direction +ve?"=TRUE, "Time offset"=0, "Amplitude offset"=0.0}, {"Start"=14402, "End"=14493, "Impulse Plane"=enum."Yaw", "Impulse Direction +ve?"=FALSE, "Time offset"=0, "Amplitude offset"=0.0}, {"Start"=14971, "End"=15063, "Impulse Plane"=enum."Yaw", "Impulse Direction +ve?"=FALSE, "Time offset"=0, "Amplitude offset"=0.0}, {"Start"=15459, "End"=15553, "Impulse Plane"=enum."Yaw", "Impulse Direction +ve?"=TRUE, "Time offset"=0, "Amplitude offset"=0.0}, {"Start"=16020, "End"=16112, "Impulse Plane"=enum."Yaw", "Impulse Direction +ve?"=FALSE, "Time offset"=0, "Amplitude offset"=0.0}, {"Start"=16530, "End"=16622, "Impulse Plane"=enum."Yaw", "Impulse Direction +ve?"=TRUE, "Time offset"=0, "Amplitude offset"=0.0}, {"Start"=17204, "End"=17295, "Impulse Plane"=enum."Yaw", "Impulse Direction +ve?"=TRUE, "Time offset"=0, "Amplitude offset"=0.0}, {"Start"=17830, "End"=17921, "Impulse Plane"=enum."Yaw", "Impulse Direction +ve?"=FALSE, "Time offset"=0, "Amplitude offset"=0.0}, {"Start"=19274, "End"=19361, "Impulse Plane"=enum."Yaw", "Impulse Direction +ve?"=FALSE, "Time offset"=0, "Amplitude offset"=0.0}, {"Start"=19884, "End"=19973, "Impulse Plane"=enum."Yaw", "Impulse Direction +ve?"=FALSE, "Time offset"=0, "Amplitude offset"=0.0}, {"Start"=20423, "End"=20518, "Impulse Plane"=enum."Yaw", "Impulse Direction +ve?"=TRUE, "Time offset"=0, "Amplitude offset"=0.0}, {"Start"=21003, "End"=21091, "Impulse Plane"=enum."Yaw", "Impulse Direction +ve?"=FALSE, "Time offset"=0, "Amplitude offset"=0.0}, {"Start"=21526, "End"=21619, "Impulse Plane"=enum."Yaw", "Impulse Direction +ve?"=FALSE, "Time offset"=0, "Amplitude offset"=0.0}, {"Start"=22032, "End"=22124, "Impulse Plane"=enum."Yaw", "Impulse Direction +ve?"=TRUE, "Time offset"=0, "Amplitude offset"=0.0}, {"Start"=22661, "End"=22752, "Impulse Plane"=enum."Yaw", "Impulse Direction +ve?"=FALSE, "Time offset"=0, "Amplitude offset"=0.0}, {"Start"=23810, "End"=23900, "Impulse Plane"=enum."Yaw", "Impulse Direction +ve?"=TRUE, "Time offset"=0, "Amplitude offset"=0.0}], "Old Impulse positions for Undo"=[], "No. Imp"=18, "Parameter Time Series"=[{"time offset"=0.0, "Offset"=0.0, "Gain"=1.0, "inverse"=FALSE, "filter data"=FALSE, "dots"=FALSE, "interpolate"=FALSE, "List 1"=1, "Color Box"=65295, "Boolean"=TRUE}, {"time offset"=0.0, "Offset"=0.0, "Gain"=1.0, "inverse"=FALSE, "filter data"=FALSE, "dots"=FALSE, "interpolate"=FALSE, "List 1"=13, "Color Box"=16777224, "Boolean"=TRUE}, {"time offset"=0.0, "Offset"=0.0, "Gain"=1.0, "inverse"=FALSE, "filter data"=FALSE, "dots"=FALSE, "interpolate"=FALSE, "List 1"=6, "Color Box"=6618880, "Boolean"=FALSE}, {"time offset"=0.0, "Offset"=0.0, "Gain"=1.0, "inverse"=FALSE, "filter data"=FALSE, "dots"=FALSE, "interpolate"=FALSE, "List 1"=14, "Color Box"=16777224, "Boolean"=FALSE}, {"time offset"=0.0, "Offset"=0.0, "Gain"=1.0, "inverse"=FALSE, "filter data"=FALSE, "dots"=FALSE, "interpolate"=FALSE, "List 1"=7, "Color Box"=6618880, "Boolean"=FALSE}, {"time offset"=0.0, "Offset"=0.0, "Gain"=1.0, "inverse"=FALSE, "filter data"=FALSE, "dots"=FALSE, "interpolate"=FALSE, "List 1"=15, "Color Box"=16777224, "Boolean"=FALSE}], "Parameter Impuls Series"=[{"Color"=4652800, "Visible"=TRUE, "Channel"=1, "Invert"=FALSE, "Desaccade"=FALSE, "Offset"=0.0, "Gain"=1.0}, {"Color"=16777224, "Visible"=TRUE, "Channel"=13, "Invert"=FALSE, "Desaccade"=FALSE, "Offset"=0.0, "Gain"=1.0}], "Experiment Parameters"={"Freq"=0.0, "Vel"=0, "Acc"=0, "Stimulus"="HIT-Lateral"}, "Autosort File"=refnum, "Data File"={"Data Channels"=array24x4503[108072 elements], "Sample Rate"=221, "Channel List"=["-", "Hz Velocity-in-Head", "-", "Hy Velocity-in-Head", "-", "Hx Velocity-in-Head", "Hl Velocity-in-Head", "Hr Velocity-in-Head", "Lx Position-in-Head", "Ly Position-in-Head", "Lz Position-in-Head", "Lx Velocity-in-Head", "Ly Velocity-in-Head", "Lz Velocity-in-Head", "Ll Velocity-in-Head", "Lr Velocity-in-Head", "-", "-", "-", "-", "-", "-", "-", "-"]}, "Experiment data path"=path "C:/Users/w.figtree/Desktop/Subject 10/Day 4", "Image data path"=path "", "LVS data path"=path "", "Raw copy path"=path "", "filename"="p00001s003e016c001t003.mat", "desaccading parameters"={"Tolerance"=0, "Acc Range"=0.0, "Sample Rate"=221, "Impulse Plane 2"=enum."Yaw", "Impulse dir"=FALSE}, "Experiment Parameters 2"={"Subject"="SE Trial Short Term", "Strain"="", "Rotation plane"="", "Experimenter"=" ", "Trial"=0.0, "Time"=0.0}, "Excel"={"Excel._Application"=refnum, "Use Excel"=TRUE, "Worksheet SINE"=refnum, "Row SINE"=0, "Worksheet TRANS"=refnum, "Row TRANS"=0}, "Session Config File"=refnum, "Autosort Parameter Set"=10, "EMA Version"="EMA 2011b", "desacc "={"Threshold 1 [Acc]"=0.0, "Threshold 2 [% of TH1]"=0, "tolerance"=0, "Search WD "=0.0, " always use TH2"=FALSE, "Range"=0.0, "Max time"=0.0, "Min time"=0.0, "Velocity Threshold"=0}, "Cycle Nr for Saccades"={"POS"=0, "NEG"=0}, "Undo Counter"=0, "History Length"=0, "Redo Counter"=0, "Histpry Position"=-1, "Raw Data File"={"Data Channels"=[], "Sample Rate"=0, "Channel List"=[]}}  # EMA 2011b Data Cluster
          # "Read LVS Data"
          n20 = call <vilib>:"Read File+ (string).vi"("count"=w119, "error in (no error)"=w116, "refnum"=w117) -> ("error out"=w114:errorcluster, "string"=w118:string, "dup refnum"=w115:refnum<file>)  [unwired: 4 in, 2 out]
          n21 = Unflatten From String(type=w119, binary string=w118) -> (value=w120:i32)  [unwired: 3 in, 2 out]
          n22 = call <vilib>:"Read File+ (string).vi"("count"=w120, "error in (no error)"=w114, "refnum"=w115) -> ("error out"=w113:errorcluster, "string"=w112:string, "dup refnum"=w108:refnum<file>)  [unwired: 4 in, 2 out]
          n23 = Bundle("\"Data File\" Cluster"=w136, "EMA 2011b Data Cluster"=w122) -> (w111:T14)  [unwired: 1 in]
          n24 = Unflatten From String(type=w111, binary string=w112, error in (no error)=w113) -> (value=w110:T14, error out=w109:errorcluster)  [unwired: 2 in, 1 out]
          n25 = Unbundle By Name(w110) -> ("EMA 2011b Data Cluster.Impulse Positions"=w133:T9, "EMA 2011b Data Cluster.No. Imp"=w132:i32, "EMA 2011b Data Cluster.Parameter Time Series"=w131:T2, "EMA 2011b Data Cluster.Parameter Impuls Series"=w130:T3, "EMA 2011b Data Cluster.Experiment Parameters"=w129:T5, "EMA 2011b Data Cluster.Autosort File"=w128:refnum<file>, "\"Data File\" Cluster"=w127:T4, "EMA 2011b Data Cluster.desaccading parameters"=w126:T12, "EMA 2011b Data Cluster.Experiment Parameters 2"=w125:T6, "EMA 2011b Data Cluster.Session Config File"=w124:refnum<file>, "EMA 2011b Data Cluster.Autosort Parameter Set"=w123:i32, "EMA 2011b Data Cluster.desacc"=w121:T15)
          n26 = Bundle By Name(cluster=w135, "Impulse Positions"=w133, "No. Imp"=w132, "Parameter Time Series"=w131, "Parameter Impuls Series"=w130, "Experiment Parameters"=w129, "Autosort File"=w128, "Data File"=w127, "desaccading parameters"=w126, "Experiment Parameters 2"=w125, "Session Config File"=w124, "Autosort Parameter Set"=w123, "desacc"=w121, "calibration name"="") -> (w134:T1)
        }
        frame "EMA 2016a" {
          w143 = T16 {"Impulse Positions"=[{"Start"=4942, "End"=5034, "Impulse Plane"=enum."Yaw", "Impulse Direction +ve?"=TRUE, "Time offset"=0, "Amplitude offset"=0.0}, {"Start"=5524, "End"=5615, "Impulse Plane"=enum."Yaw", "Impulse Direction +ve?"=FALSE, "Time offset"=0, "Amplitude offset"=0.0}, {"Start"=6320, "End"=6414, "Impulse Plane"=enum."Yaw", "Impulse Direction +ve?"=FALSE, "Time offset"=0, "Amplitude offset"=0.0}, {"Start"=6789, "End"=6880, "Impulse Plane"=enum."Yaw", "Impulse Direction +ve?"=TRUE, "Time offset"=0, "Amplitude offset"=0.0}, {"Start"=7275, "End"=7365, "Impulse Plane"=enum."Yaw", "Impulse Direction +ve?"=FALSE, "Time offset"=0, "Amplitude offset"=0.0}, {"Start"=7765, "End"=7854, "Impulse Plane"=enum."Yaw", "Impulse Direction +ve?"=FALSE, "Time offset"=0, "Amplitude offset"=0.0}, {"Start"=8262, "End"=8354, "Impulse Plane"=enum."Yaw", "Impulse Direction +ve?"=TRUE, "Time offset"=0, "Amplitude offset"=0.0}, {"Start"=9102, "End"=9192, "Impulse Plane"=enum."Yaw", "Impulse Direction +ve?"=TRUE, "Time offset"=0, "Amplitude offset"=0.0}, {"Start"=9641, "End"=9736, "Impulse Plane"=enum."Yaw", "Impulse Direction +ve?"=FALSE, "Time offset"=0, "Amplitude offset"=0.0}, {"Start"=10150, "End"=10242, "Impulse Plane"=enum."Yaw", "Impulse Direction +ve?"=FALSE, "Time offset"=0, "Amplitude offset"=0.0}, {"Start"=10613, "End"=10703, "Impulse Plane"=enum."Yaw", "Impulse Direction +ve?"=TRUE, "Time offset"=0, "Amplitude offset"=0.0}, {"Start"=11147, "End"=11237, "Impulse Plane"=enum."Yaw", "Impulse Direction +ve?"=TRUE, "Time offset"=0, "Amplitude offset"=0.0}, {"Start"=11689, "End"=11781, "Impulse Plane"=enum."Yaw", "Impulse Direction +ve?"=TRUE, "Time offset"=0, "Amplitude offset"=0.0}, {"Start"=12321, "End"=12416, "Impulse Plane"=enum."Yaw", "Impulse Direction +ve?"=FALSE, "Time offset"=0, "Amplitude offset"=0.0}, {"Start"=12810, "End"=12901, "Impulse Plane"=enum."Yaw", "Impulse Direction +ve?"=FALSE, "Time offset"=0, "Amplitude offset"=0.0}, {"Start"=13306, "End"=13397, "Impulse Plane"=enum."Yaw", "Impulse Direction +ve?"=FALSE, "Time offset"=0, "Amplitude offset"=0.0}, {"Start"=13888, "End"=13980, "Impulse Plane"=enum."Yaw", "Impulse Direction +ve?"=TRUE, "Time offset"=0, "Amplitude offset"=0.0}, {"Start"=14402, "End"=14493, "Impulse Plane"=enum."Yaw", "Impulse Direction +ve?"=FALSE, "Time offset"=0, "Amplitude offset"=0.0}, {"Start"=14971, "End"=15063, "Impulse Plane"=enum."Yaw", "Impulse Direction +ve?"=FALSE, "Time offset"=0, "Amplitude offset"=0.0}, {"Start"=15459, "End"=15553, "Impulse Plane"=enum."Yaw", "Impulse Direction +ve?"=TRUE, "Time offset"=0, "Amplitude offset"=0.0}, {"Start"=16020, "End"=16112, "Impulse Plane"=enum."Yaw", "Impulse Direction +ve?"=FALSE, "Time offset"=0, "Amplitude offset"=0.0}, {"Start"=16530, "End"=16622, "Impulse Plane"=enum."Yaw", "Impulse Direction +ve?"=TRUE, "Time offset"=0, "Amplitude offset"=0.0}, {"Start"=17204, "End"=17295, "Impulse Plane"=enum."Yaw", "Impulse Direction +ve?"=TRUE, "Time offset"=0, "Amplitude offset"=0.0}, {"Start"=17830, "End"=17921, "Impulse Plane"=enum."Yaw", "Impulse Direction +ve?"=FALSE, "Time offset"=0, "Amplitude offset"=0.0}, {"Start"=19274, "End"=19361, "Impulse Plane"=enum."Yaw", "Impulse Direction +ve?"=FALSE, "Time offset"=0, "Amplitude offset"=0.0}, {"Start"=19884, "End"=19973, "Impulse Plane"=enum."Yaw", "Impulse Direction +ve?"=FALSE, "Time offset"=0, "Amplitude offset"=0.0}, {"Start"=20423, "End"=20518, "Impulse Plane"=enum."Yaw", "Impulse Direction +ve?"=TRUE, "Time offset"=0, "Amplitude offset"=0.0}, {"Start"=21003, "End"=21091, "Impulse Plane"=enum."Yaw", "Impulse Direction +ve?"=FALSE, "Time offset"=0, "Amplitude offset"=0.0}, {"Start"=21526, "End"=21619, "Impulse Plane"=enum."Yaw", "Impulse Direction +ve?"=FALSE, "Time offset"=0, "Amplitude offset"=0.0}, {"Start"=22032, "End"=22124, "Impulse Plane"=enum."Yaw", "Impulse Direction +ve?"=TRUE, "Time offset"=0, "Amplitude offset"=0.0}, {"Start"=22661, "End"=22752, "Impulse Plane"=enum."Yaw", "Impulse Direction +ve?"=FALSE, "Time offset"=0, "Amplitude offset"=0.0}, {"Start"=23810, "End"=23900, "Impulse Plane"=enum."Yaw", "Impulse Direction +ve?"=TRUE, "Time offset"=0, "Amplitude offset"=0.0}], "Old Impulse positions for Undo"=[], "No. Imp"=18, "Parameter Time Series"=[{"time offset"=0.0, "Offset"=0.0, "Gain"=1.0, "inverse"=FALSE, "filter data"=FALSE, "dots"=FALSE, "interpolate"=FALSE, "List 1"=1, "Color Box"=65295, "Boolean"=TRUE}, {"time offset"=0.0, "Offset"=0.0, "Gain"=1.0, "inverse"=FALSE, "filter data"=FALSE, "dots"=FALSE, "interpolate"=FALSE, "List 1"=13, "Color Box"=16777224, "Boolean"=TRUE}, {"time offset"=0.0, "Offset"=0.0, "Gain"=1.0, "inverse"=FALSE, "filter data"=FALSE, "dots"=FALSE, "interpolate"=FALSE, "List 1"=6, "Color Box"=6618880, "Boolean"=FALSE}, {"time offset"=0.0, "Offset"=0.0, "Gain"=1.0, "inverse"=FALSE, "filter data"=FALSE, "dots"=FALSE, "interpolate"=FALSE, "List 1"=14, "Color Box"=16777224, "Boolean"=FALSE}, {"time offset"=0.0, "Offset"=0.0, "Gain"=1.0, "inverse"=FALSE, "filter data"=FALSE, "dots"=FALSE, "interpolate"=FALSE, "List 1"=7, "Color Box"=6618880, "Boolean"=FALSE}, {"time offset"=0.0, "Offset"=0.0, "Gain"=1.0, "inverse"=FALSE, "filter data"=FALSE, "dots"=FALSE, "interpolate"=FALSE, "List 1"=15, "Color Box"=16777224, "Boolean"=FALSE}], "Parameter Impuls Series"=[{"Color"=4652800, "Visible"=TRUE, "Channel"=1, "Invert"=FALSE, "Desaccade"=FALSE, "Offset"=0.0, "Gain"=1.0}, {"Color"=16777224, "Visible"=TRUE, "Channel"=13, "Invert"=FALSE, "Desaccade"=FALSE, "Offset"=0.0, "Gain"=1.0}], "Experiment Parameters"={"Freq"=0.0, "Vel"=0, "Acc"=0, "Stimulus"="HIT-Lateral"}, "Autosort File"=refnum, "Data File"={"Data Channels"=array24x4503[108072 elements], "Sample Rate"=221, "Channel List"=["-", "Hz Velocity-in-Head", "-", "Hy Velocity-in-Head", "-", "Hx Velocity-in-Head", "Hl Velocity-in-Head", "Hr Velocity-in-Head", "Lx Position-in-Head", "Ly Position-in-Head", "Lz Position-in-Head", "Lx Velocity-in-Head", "Ly Velocity-in-Head", "Lz Velocity-in-Head", "Ll Velocity-in-Head", "Lr Velocity-in-Head", "-", "-", "-", "-", "-", "-", "-", "-"]}, "Experiment data path"=path "C:/Users/w.figtree/Desktop/Subject 10/Day 4", "Image data path"=path "", "LVS data path"=path "", "Raw copy path"=path "", "filename"="p00001s003e016c001t003.mat", "desaccading parameters"={"Tolerance"=0, "Acc Range"=0.0, "Sample Rate"=221, "Impulse Plane 2"=enum."Yaw", "Impulse dir"=FALSE}, "Experiment Parameters 2"={"Subject"="SE Trial Short Term", "Strain"="", "Rotation plane"="", "Experimenter"=" ", "Trial"=0.0, "Time"=0.0}, "Excel"={"Excel._Application"=refnum, "Use Excel"=TRUE, "Worksheet SINE"=refnum, "Row SINE"=0, "Worksheet TRANS"=refnum, "Row TRANS"=0}, "Session Config File"=refnum, "Autosort Parameter Set"=10, "EMA Version"="EMA 2011b", "desacc "={"Threshold 1 [Acc]"=0.0, "Threshold 2 [% of TH1]"=0, "tolerance"=0, "Search WD "=0.0, " always use TH2"=FALSE, "Range"=0.0, "Max time"=0.0, "Min time"=0.0, "Velocity Threshold"=0}, "Cycle Nr for Saccades"={"POS"=0, "NEG"=0}, "Undo Counter"=0, "History Length"=0, "Redo Counter"=0, "Histpry Position"=-1, "Raw Data File"={"Data Channels"=[], "Sample Rate"=0, "Channel List"=[]}, "calibration name"="p00001s003_calib.mat"}  # EMA 2016a Data Cluster
          # "Read LVS Data"
          n27 = Bundle("\"Data File\" Cluster"=w159, "EMA 2016a Data Cluster"=w143) -> (w138:T17)  [unwired: 1 in]
          n28 = Read from Binary File(5:w138, 8:w141, 11:w142) -> (0:w139:errorcluster, 2:w137:T17, 3:w140:refnum<file>)  [unwired: 3 in, 1 out]
          n29 = Unbundle By Name(w137) -> ("EMA 2016a Data Cluster.Impulse Positions"=w156:T9, "EMA 2016a Data Cluster.No. Imp"=w155:i32, "EMA 2016a Data Cluster.Parameter Time Series"=w154:T2, "EMA 2016a Data Cluster.Parameter Impuls Series"=w153:T3, "EMA 2016a Data Cluster.Experiment Parameters"=w152:T5, "EMA 2016a Data Cluster.Autosort File"=w151:refnum<file>, "\"Data File\" Cluster"=w150:T4, "EMA 2016a Data Cluster.desaccading parameters"=w149:T12, "EMA 2016a Data Cluster.Experiment Parameters 2"=w148:T6, "EMA 2016a Data Cluster.Session Config File"=w147:refnum<file>, "EMA 2016a Data Cluster.Autosort Parameter Set"=w146:i32, "EMA 2016a Data Cluster.desacc"=w145:T15, "EMA 2016a Data Cluster.calibration name"=w144:string)
          n30 = Bundle By Name(cluster=w158, "Impulse Positions"=w156, "No. Imp"=w155, "Parameter Time Series"=w154, "Parameter Impuls Series"=w153, "Experiment Parameters"=w152, "Autosort File"=w151, "Data File"=w150, "desaccading parameters"=w149, "Experiment Parameters 2"=w148, "Session Config File"=w147, "Autosort Parameter Set"=w146, "desacc"=w145, "calibration name"=w144) -> (w157:T1)
        }
        frame "EMA 2017a" {
          w162 = T18 {"Impulse Positions"=[], "No. Imp"=0, "Parameter Time Series"=[], "Parameter Impuls Series"=[], "Experiment Parameters"={"Freq"=0.0, "Vel"=0, "Acc"=0, "Stimulus"=""}, "Autosort File"=refnum, "Data File"={"Data Channels"=[], "Sample Rate"=0, "Channel List"=[]}, "Experiment data path"=path "/Macintosh HD/Users/patrick/Studium/Diploma Thesis/Data Analysis", "Image data path"=path "/Macintosh HD/Users/patrick/Studium/Diploma Thesis/Data Analysis", "LVS data path"=path "/Macintosh HD/Users/patrick/Studium/Diploma Thesis/Data Analysis", "Raw copy path"=path "/Macintosh HD/Users/patrick/Studium/Diploma Thesis/Data Analysis", "filename"="No file selected", "desaccading parameters"={"Tolerance"=0, "Acc Range"=0.0, "Sample Rate"=0, "Impulse Plane 2"=enum."Other", "Impulse dir"=FALSE}, "Experiment Parameters 2"={"Subject"="", "Strain"="", "Rotation plane"="", "Experimenter"="", "Trial"=0.0, "Time"=0.0}, "Excel"={"Excel._Application"=refnum, "Use Excel"=FALSE, "Worksheet SINE"=refnum, "Row SINE"=0, "Worksheet TRANS"=refnum, "Row TRANS"=0}, "Session Config File"=refnum, "Autosort Parameter Set"=1, "EMA Version"="", "desacc "={"Threshold 1 [Acc]"=7000.0, "Threshold 2 [% of TH1]"=60, "tolerance"=3, "Search WD "=0.1, " always use TH2"=FALSE, "Range"=2.0, "Max time"=120.0, "Min time"=20.0, "Velocity Threshold"=150}, "Cycle Nr for Saccades"={"POS"=0, "NEG"=0}, "calibration name"="No file selected"}  # EMA 2017a Data Cluster
          n31 = Read from Binary File(5:w162, 8:w181, 11:w182) -> (0:w163:errorcluster, 2:w180:T18, 3:w164:refnum<file>)  [unwired: 3 in, 1 out]
          n32 = Unbundle By Name(w180) -> ("Impulse Positions"=w177:T9, "No. Imp"=w176:i32, "Parameter Time Series"=w175:T2, "Parameter Impuls Series"=w174:T3, "Experiment Parameters"=w173:T5, "Autosort File"=w172:refnum<file>, "Data File"=w171:T4, "desaccading parameters"=w170:T12, "Experiment Parameters 2"=w169:T6, "Session Config File"=w168:refnum<file>, "Autosort Parameter Set"=w167:i32, "desacc"=w166:T15, "calibration name"=w165:string, "Experiment data path"=w161:path, "filename"=w160:string)
          n33 = Bundle By Name(cluster=w179, "Impulse Positions"=w177, "No. Imp"=w176, "Parameter Time Series"=w175, "Parameter Impuls Series"=w174, "Experiment Parameters"=w173, "Autosort File"=w172, "Data File"=w171, "desaccading parameters"=w170, "Experiment Parameters 2"=w169, "Session Config File"=w168, "Autosort Parameter Set"=w167, "desacc"=w166, "calibration name"=w165, "Experiment data path"=w161, "filename"=w160) -> (w178:T1)
        }
      }
      n34 = case shown="No Error" w12 {
        selector: w12 -> [w24 w42]
        tunnel: w11 -> [w27 _]
        tunnel: w10 -> [w25 w43]
        tunnel: w9 -> [w31 _]
        tunnel: [w26 w43] -> w8
        tunnel: [w24 w42] -> w7
        frame No Error {
          # "Manage working directory."
          n35 = Strip Path(path=w31) -> (stripped path=w28:path, name=w29:string)
          n36 = Strip Path(path=w28) -> (name=w30:string)  [unwired: 1 out]
          n37 = case shown="\"EMA-Configuration\"" w30 {
            tunnel: w29 -> [w33 w39 _]
            tunnel: w28 -> [w34 _ _]
            tunnel: w27 -> [w35 w40 w41]
            tunnel: [w32 w38 w41] -> w26
            tunnel: w25 -> [_ w37 _]
            frame Default {
              # "Regular LVS directory. Just set the name and directory based on this file."
              n38 = Bundle By Name(cluster=w35, "Experiment data path"=w34, "filename"=w33) -> (w32:T1)
            }
            frame "tmp_batch_lvs" {
              # "Temporary LVS file. Keep directory from function input but change file name."
              n39 = Unbundle By Name(w37) -> ("Experiment data path"=w36:path)
              n40 = Bundle By Name(cluster=w40, "filename"=w39, "Experiment data path"=w36) -> (w38:T1)
            }
            frame "EMA-Configuration" {
              # "Session LVS file. Grab filename and directory from loaded LVS file."
            }
          }
        }
        frame Error {
          # "Discard any changes on error."
        }
      }
      n41 = Close File(refnum=w17) -> (path=w15:path, error out=w16:errorcluster)  [unwired: 1 in]
      n42 = call <vilib>:"Clear Errors.vi"("error in (no error)"=w16) -> ()  [unwired: 5 in, 2 out]
    }
    frame Error {
    }
  }
  "error out" <- w3
  "LVS Data (out)" <- w2
  "Path (out)" <- w4
